vi "California Instruments iX Series Acquire Measurements.vi"() -> ()   [LabVIEW 2010]
doc: "Demonstrates reading Current, Voltage and Power measurements for each phase."
uses:
  <instrlib>/California Instruments iX Series/Public/Data/Read Single Voltage Measurement.vi
  <instrlib>/California Instruments iX Series/Public/Data/Read Single Current Measurement.vi
  <instrlib>/California Instruments iX Series/California Instruments iX Series.lvlib
panel:
  in  "Stop":bool
  out "Power Measurement":dbl[](array[numeric])
  out "Current Measurement":dbl[](array[numeric])
  out "Voltage Measurement":dbl[](array[numeric])
  in  "Voltage Measurement Type (0:DC)":u16(ring) items=["DC", "AC", "AC+DC", "Voltage Harmonic THD"]
  in  "Current Measurement Type (0:DC)":u16(ring) items=["DC", "AC", "AC+DC", "Crest Factor", "Current Harmonic THD", "Neutral DC", "Neutral AC", "Neutral ACDC"]
  in  "Power Measurement Type (0: DC Power)":u16(ring) items=["DC Power", "Real Power", "Apparent Power", "Reactive Power", "Power Factor", "Total Power"]
  in  "Serial Configuration":cluster{"Baud Rate":u32, "Flow Control":u16}={"Baud Rate"=460800, "Flow Control"=0} {"Flow Control" items=["None", "XON/XOFF", "RTS/CTS", "XON/XOFF & RTS/CTS", "DTR/DSR", "XON/XOFF & DTR/DSR"]; "Baud Rate" items=["9600"=9600, "19200"=19200, "38400"=38400, "57600"=57600, "115200"=115200, "230400"=230400, "460800"=460800]}
  in  "VISA resource name":refnum<visa-resource-name>
  # "(c) 2009 National Instruments.  ALL RIGHTS RESERVED."
  # "Measurements"
  # "Measurement Type"
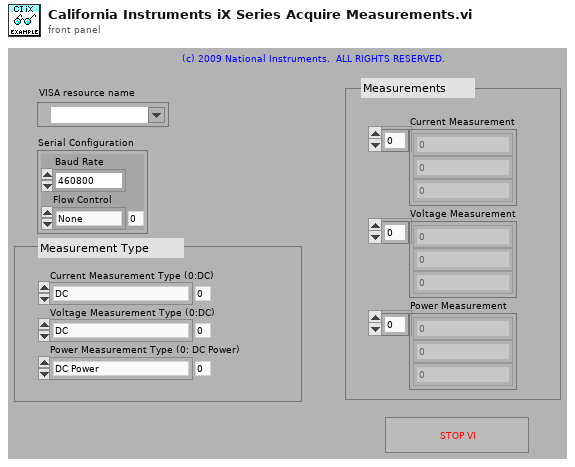
[diagram p1: front panel]
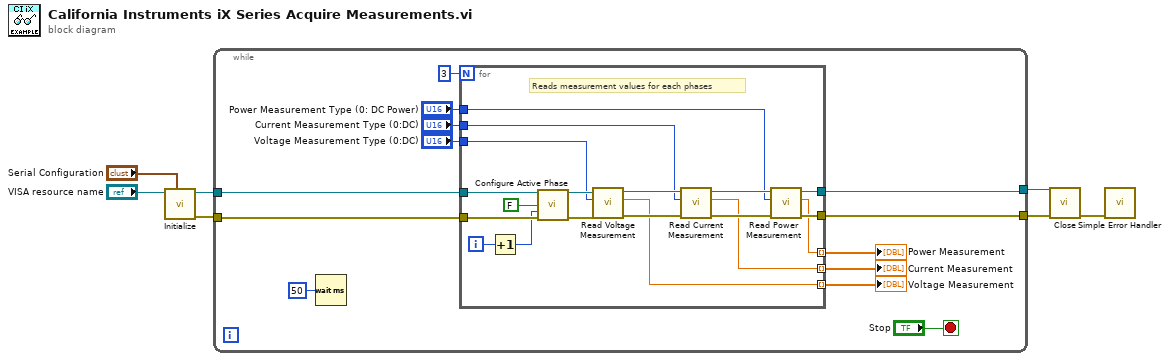
[diagram p0: block diagram]
diagram:
  n1 = call <instrlib>:"Initialize.vi"("Serial Configuration"="Serial Configuration", "VISA resource name"="VISA resource name") -> ("error out"=w1:errorcluster, "VISA resource name out"=w2:refnum<visa-resource-name>)  [unwired: 8 in]
  n2 = while {
    tunnel: [w20] -> w4
    tunnel: [w19] -> w5
    tunnel: w2 -> [w17]
    tunnel: w1 -> [w16]
    stop <- "Stop" stop-if-true
    n3 = Wait (ms)(milliseconds to wait=u32 50) -> ()  [unwired: 1 out]
    n4 = for {
      N: 3 -> [_]
      tunnel: [w35] -> w20
      tunnel: [w34] -> w19
      tunnel: w17 -> [w33]
      tunnel: w16 -> [w32]
      tunnel: "Power Measurement Type (0: DC Power)" -> [w27]
      tunnel: "Current Measurement Type (0:DC)" -> [w26]
      tunnel: "Voltage Measurement Type (0:DC)" -> [w25]
      tunnel: [w24] -> w11 mode=indexing
      tunnel: [w23] -> w10 mode=indexing
      tunnel: [w22] -> w9 mode=indexing
      i -> [w28]
      # "Reads measurement values for each phases"
      n5 = Increment(x=w28) -> (x+1=w29:i32)
      n6 = call <instrlib>:"Configure Active Phase.vi"("VISA resource name"=w33, "Enable Coupling (Enabled)"=FALSE ("Enabled Coupling (Enabled)"), "Active Phase (1:Phase 1)"=w29, "error in (no error)"=w32) -> ("VISA resource name out"=w31:refnum<visa-resource-name>, "error out"=w30:errorcluster)  [unwired: 10 in]
      n7 = call-poly <instrlib>:"Read Voltage Measurement.vi"("error in (no error)"=w30, "Single Voltage Measurement Type (0:DC)"=w25, "VISA resource name"=w31) -> ("error out"=w38:errorcluster, "Voltage Measurement"=w24:dbl, "VISA resource name out"=w39:refnum<visa-resource-name>)  [unwired: 6 in]
      n8 = call-poly <instrlib>:"Read Current Measurement.vi"("error in (no error)"=w38, "Single Current Measurement Type (0:DC)"=w26, "VISA resource name"=w39) -> ("error out"=w37:errorcluster, "Current Measurement"=w23:dbl, "VISA resource name out"=w36:refnum<visa-resource-name>)  [unwired: 6 in]
      n9 = call <instrlib>:"Read Power Measurement.vi"("error in (no error)"=w37, "Power Measurement Type (0: DC Power)"=w27, "VISA resource name"=w36) -> ("error out"=w34:errorcluster, "Power Measurement"=w22:dbl, "VISA resource name out"=w35:refnum<visa-resource-name>)  [unwired: 6 in]
    }
    "Voltage Measurement" <- w11
    "Current Measurement" <- w10
    "Power Measurement" <- w9
  }
  n10 = call <instrlib>:"Close.vi"("error in (no error)"=w5, "VISA resource name"=w4) -> ("error out"=w3:errorcluster)  [unwired: 9 in]
  n11 = call <vilib>:"Simple Error Handler.vi"("error in (no error)"=w3) -> ()  [unwired: 4 in, 5 out]
